vi "Find Window.vi"(8 "error in (no error)":errorcluster, 11 "Window Title (Callers Window)":string) -> (0 "error out":errorcluster, 3 "Window Handle":refnum<k24>)   [LabVIEW 2011, in "TaskbarProgressAPI.lvlib"]
doc: "Find a Window based on it's name and returns it's Handle packed in a .Net IntPtr object.\n\nPlease see the 'LabVIEW Taskbar Progress Bar API Example.vi' in the NI Example finder for details on how to use this VI."
uses:
  TaskbarProgressAPI.lvlib
  kernel32.dll
  User32.dll
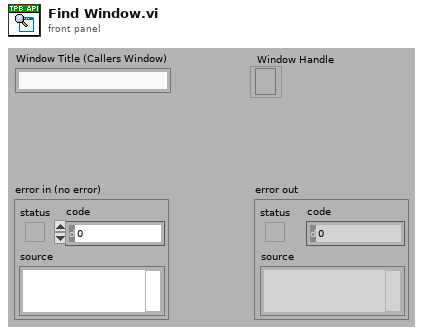
[diagram p1: front panel]
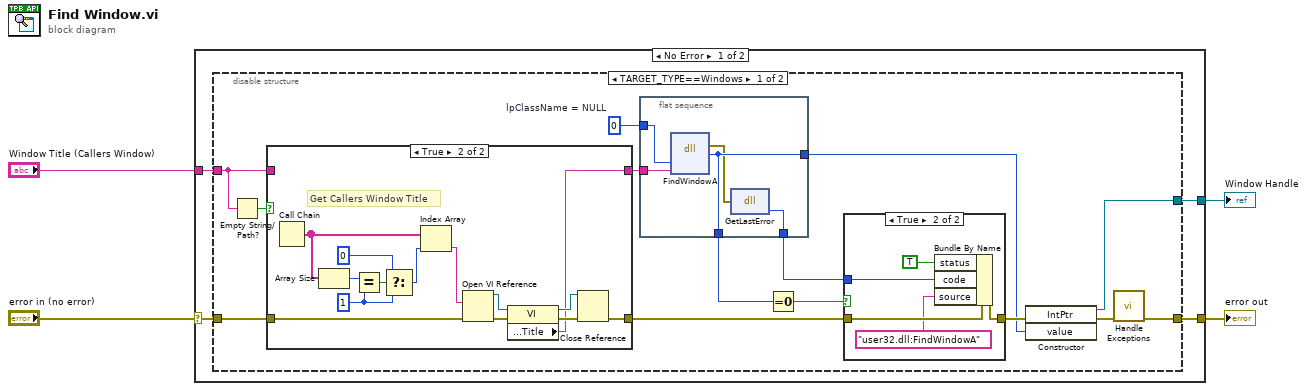
[diagram p0: block diagram]
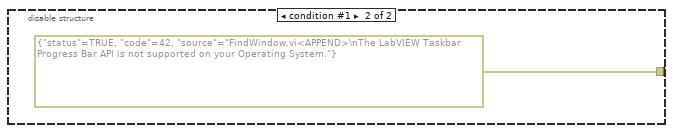
[diagram p4: hidden frame]
diagram:
  n1 = case shown="No Error" "error in (no error)" {
    selector: "error in (no error)" -> [w7 w51]
    tunnel: [w6 w51] -> w3
    tunnel: "Window Title (Callers Window)" -> [w8 _]
    tunnel: [w5 _] -> w1
    frame No Error {
      n2 = disable-structure shown="TARGET_TYPE==Windows" {
        disable-tunnel: w8 -> [w19 _]
        disable-tunnel: w7 -> [w17 _]
        disable-tunnel: [w12 errorcluster {"status"=TRUE, "code"=42, "source"="FindWindow.vi<APPEND>\nThe LabVIEW Taskbar Progress Bar API is not supported on your Operating System."} ("error out")] -> w6
        disable-tunnel: [w14 _] -> w5
        frame condition #0 (active) {
          w21 = u32 0  # lpClassName = NULL
          n3 = Empty String/Path?(string/path=w19) -> (empty?=w20:bool)
          n4 = case shown="True" w20 {
            tunnel: w19 -> [w29 _]
            tunnel: [w29 w31] -> w18
            tunnel: w17 -> [w28 w36]
            tunnel: [w28 w30] -> w16
            frame False {
            }
            frame True {
              w40 = 1 ("y")
              # "Get Callers Window Title"
              n5 = Call Chain() -> (call chain=w43:string[])
              n6 = Array Size(array=w43) -> (size(s)=w42:i32)
              n7 = Equal?(x=w42, y=w40) -> (x = y?=w41:bool)
              n8 = Select(t=0, s=w41, f=w40) -> (s? t:f=w38:i32)
              n9 = Index Array(array=w43, index=w38) -> (element=w37:string)
              n10 = Open VI Reference(vi path=w37, error in (no error)=w36) -> (vi reference=w34:refnum<vi>, error out=w35:errorcluster)  [unwired: 4 in]
              n11 = property class="VI"(reference=w34, error in=w35) -> (reference out=w32:refnum<vi>, error out=w33:errorcluster, "Front Panel.Title"=w31:string)
              n12 = Close Reference(reference=w32, error in (no error)=w33) -> (error out=w30:errorcluster)
            }
          }
          n13 = flat-sequence {
            tunnel: w21 -> [w27]
            tunnel: w18 -> [w26]
            tunnel: [w25] -> w10
            tunnel: [w25] -> w11
            tunnel: [w24] -> w9
            frame #0 {
              n14 = dll-call lib="user32.dll" fn="FindWindowA"("lpClassName"=w27, "lpWindowName"=w26) -> (error out=w23:errorcluster, "return type"=w25:i64)  [unwired: 5 in, 1 out]
              n15 = dll-call lib="kernel32.dll" fn="GetLastError"(error in=w23) -> ("return type"=w24:i32)  [unwired: 2 in, 2 out]
            }
          }
          n16 = Equal To 0?(x=w10) -> (x = 0?=w22:bool)
          n17 = case shown="True" w22 {
            tunnel: [w44 w48] -> w15
            tunnel: w16 -> [w44 w49]
            tunnel: w9 -> [_ w45]
            frame False {
            }
            frame True {
              n18 = Bundle By Name(cluster=w49, "status"=TRUE, "code"=w45, "source"="user32.dll:FindWindowA" ("Function")) -> (w48:errorcluster)
            }
          }
          n19 = constructor class="IntPtr"(error in=w15, "value"=w11) -> (reference out=w14:refnum<k24>, error out=w13:errorcluster)  [unwired: 2 in, 2 out]
          n20 = call "Handle Exceptions.vi"("error in (no error)"=w13) -> ("error out"=w12:errorcluster)  [unwired: 10 in]
        }
        frame condition #1 {
        }
      }
    }
    frame Error {
    }
  }
  "error out" <- w3
  "Window Handle" <- w1
